vi "Check Index Ramp.vi"(11 "Plot Indices":i32[](array[numeric])) -> (8 "Ramp Type":enum16{"increasing", "decreasing"}(ring), 10 "Plot Indices (dup)":i32[](array[numeric]), 12 "Contiguous?":bool)   [LabVIEW 2019]
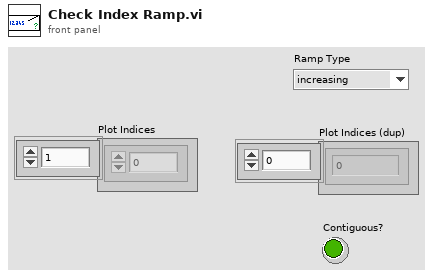
[diagram p1: front panel]
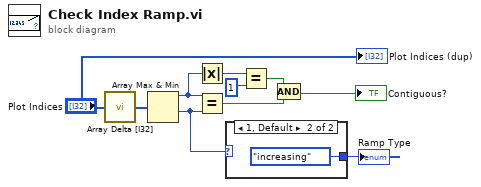
[diagram p0: block diagram]
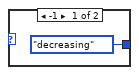
[diagram p2: hidden frame]
diagram:
  n1 = call "Array Delta [I32].vi"("Array in"="Plot Indices") -> ("Array Delta out"=w10:i32[])  [unwired: 8 in]
  n2 = Array Max & Min(array=w10) -> (max value=w5:i32, min value=w8:i32)  [unwired: 2 out]
  n3 = Absolute Value(x=w5) -> (abs(x)=w4:i32)
  n4 = Equal?(x=w5, y=w8) -> (x = y?=w9:bool)
  n5 = case shown="1, Default" w8 {
    tunnel: [enum16{"increasing", "decreasing"}."decreasing" ("Ramp Type") enum16{"increasing", "decreasing"}."increasing" ("Ramp Type")] -> w6
    frame -1 {
    }
    frame 1, Default {
    }
  }
  "Ramp Type" <- w6
  n6 = Equal?(x=w4, y=1) -> (x = y?=w1:bool)
  n7 = Compound Arithmetic op=AND(w1, w9) -> (→"Contiguous?":bool)
  "Plot Indices (dup)" <- "Plot Indices"
